vi "controllerView.vi"(10 "UserEvents in":refnum<class "UserEvents.lvclass">) -> ()   [LabVIEW 2013, in "FAMTViews.lvlib"]
uses:
  FAMTViews.lvlib
  UserEvents/UserEvents.lvclass
  Typedefs/ForceDemand.ctl
  UserEvents/UserEvents.lvclass/UserEvents.ctl
  Typedefs/StateSelector.ctl
  Typedefs/FAMTTypedefs.lvlib
panel:
  out "Force Error":T1 min=-888.0 max=888.0 format="%.2f"
  out "Force Demand":T1 min=-888.0 max=888.0 format="%.2f"
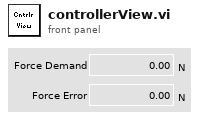
[diagram p1: front panel]
types:
  T1 = typedef "FAMTTypedefs.lvlib/ForceDemand.ctl" = dbl[unit]
  T2 = typedef "FAMTTypedefs.lvlib/PubDataEvents.ctl" = cluster{"State":refnum<user-event>, "ErrorCode":refnum<user-event>, "OutputData":refnum<user-event>, "InputData":refnum<user-event>, "ControllerData":refnum<user-event>, "TestStatus":refnum<user-event>, "LogPath":refnum<user-event>, "StiffnessData":refnum<user-event>}
  T3 = cluster{"Event Registration Refnum":refnum<event-registration>, "Event Registration Refnum":refnum<event-registration>}
  T4 = typedef "FAMTTypedefs.lvlib/StateSelector.ctl" = enum16{"EndingCycleState", "FaultState", "InteractiveMotionState", "MovingToNewForceState", "OffState", "PausingState", "StandbyState", "StoppedState"}
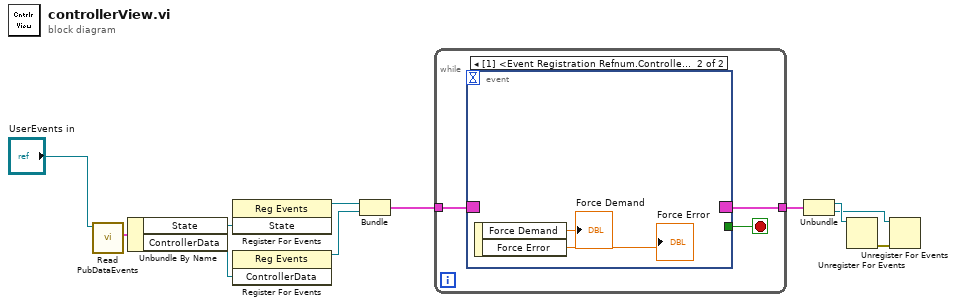
[diagram p0: block diagram]
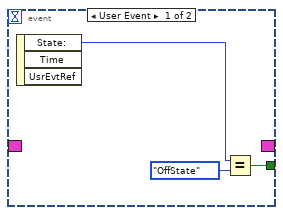
[diagram p2: hidden frame]
diagram:
  n1 = call "Read PubDataEvents.vi"("UserEvents in"="UserEvents in") -> ("PubDataEvents"=w7:T2)  [unwired: 9 in, 1 out]
  n2 = Unbundle By Name(w7) -> ("State"=w8:refnum<user-event>, "ControllerData"=w10:refnum<user-event>)
  n3 = register-events(w8) -> (reference out=w9:refnum<event-registration>)  [unwired: 2 in, 1 out]
  n4 = register-events(w10) -> (reference out=w11:refnum<event-registration>)  [unwired: 2 in, 1 out]
  n5 = Bundle("Event Registration Refnum"=w9, "Event Registration Refnum"=w11) -> (w6:T3)  [unwired: 1 in]
  n6 = while {
    tunnel: w6 -> [w14]
    tunnel: [w13] -> w5
    stop <- w12 stop-if-true
    n7 = event shown="[1] <Event Registration Refnum.ControllerData>: User Event" {
      selector: w14 -> [_ _]
      dyn-events: [_ _] -> w13
      timeout: _ -> [_ _]
      tunnel: [w15 _] -> w12
      event User Event {
        n8 = event-data() -> ("State:"=w16:T4)  [unwired: 1 in, 2 out]
        n9 = Equal?(x=w16, y=StateSelector."OffState") -> (x = y?=w15:bool)
      }
      event User Event {
        n10 = event-data() -> ("Force Demand"=→"Force Demand":T1, "Force Error"=→"Force Error":T1)  [unwired: 1 in]
      }
    }
  }
  n11 = Unbundle(w5) -> ("Event Registration Refnum"=w4:refnum<event-registration>, "Event Registration Refnum"=w2:refnum<event-registration>)
  n12 = Unregister For Events(event registration refnum=w4) -> (error out=w3:errorcluster)  [unwired: 1 in]
  n13 = Unregister For Events(event registration refnum=w2, error in=w3) -> ()  [unwired: 1 out]
